vi "song_processing1.vi"() -> ()   [LabVIEW 2019]
panel:
  out "1/x":dbl
  out "x*y":dbl
  out "data":waveform(dbl)[](array[waveform])
  in  "path":path
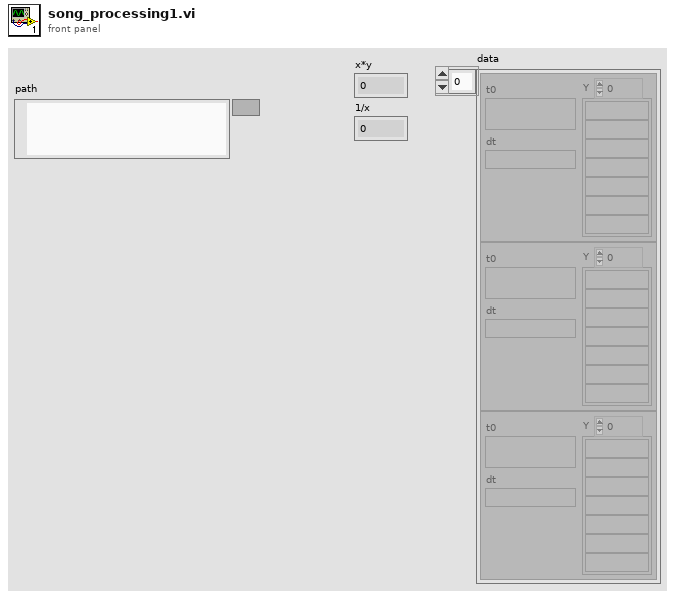
[diagram p1: front panel]
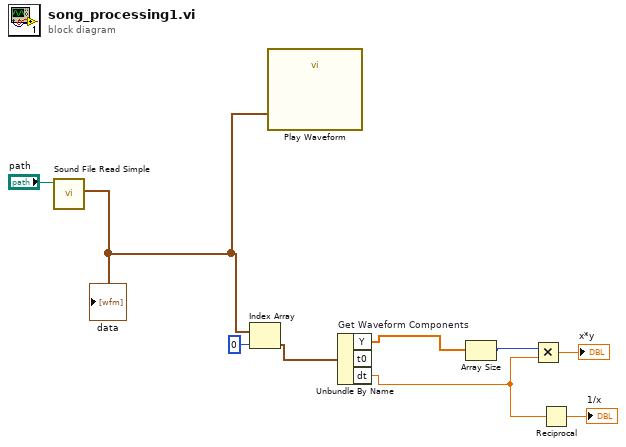
[diagram p0: block diagram]
diagram:
  n1 = call <vilib>:"Sound File Read Simple.vi"("path"="path") -> ("data"=w7:waveform(dbl)[])  [unwired: 7 in, 3 out]
  "data" <- w7
  n2 = Index Array(array=w7, index=0) -> (element=w6:waveform(dbl))
  n3 = call "Play Waveform"("Data"=w7) -> ()  [unwired: 18 in, 1 out]
  n4 = Unbundle By Name "Get Waveform Components"(w6) -> ("Y"=w5:dbl[], "dt"=w2:dbl)  [unwired: 1 out]
  n5 = Array Size(array=w5) -> (size(s)=w4:i32)
  n6 = Multiply(x=w4, y=w2) -> (x*y=→"x*y":dbl)
  n7 = Reciprocal(x=w2) -> (1/x=→"1/x":dbl)
